vi "Telnet_Init_Challenge_v2.vi"(2 "Max_trials":i32=10, 3 "Address":string="192.168.10.152") -> (0 "connection ID out":refnum<k5>, 1 "telnet_status":bool)   [LabVIEW 2018]
panel:
  out "conn_status":bool
  out "string out":string
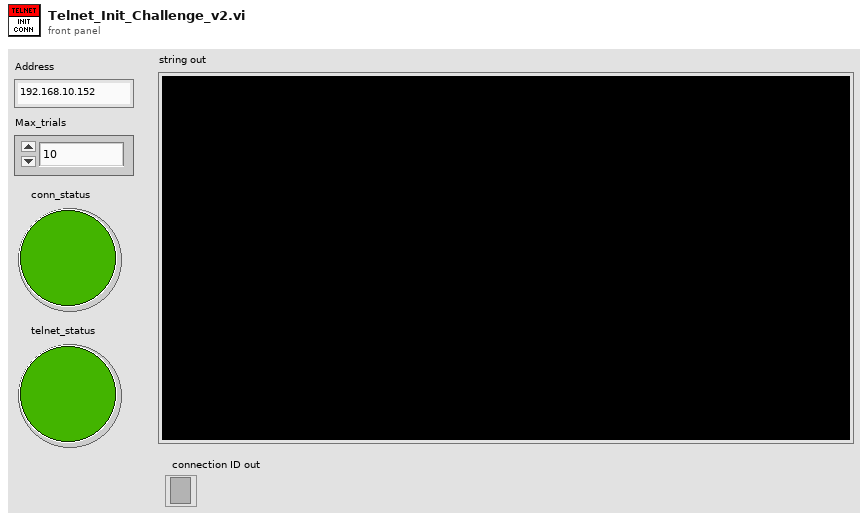
[diagram p1: front panel]
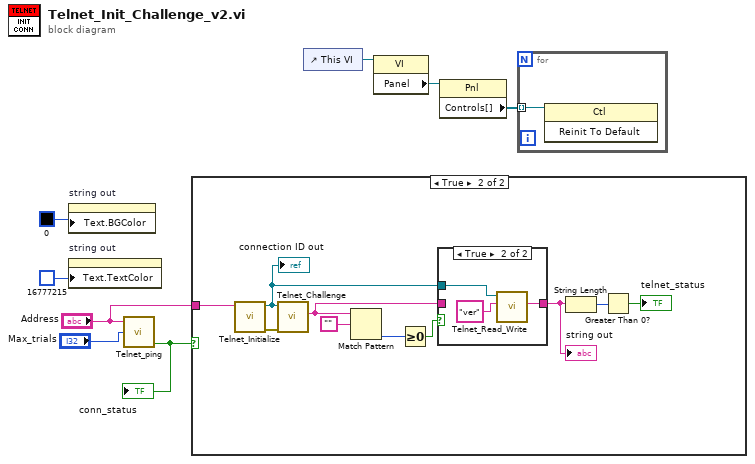
[diagram p0: block diagram]
diagram:
  n1 = property on="string out" class="Str"("Text.BGColor"=u32 0) -> ()  [unwired: 2 in, 2 out]
  n2 = property on="string out" class="Str"("Text.TextColor"=u32 16777215) -> ()  [unwired: 2 in, 2 out]
  n3 = call "Telnet_ping.vi"("Max_trials"="Max_trials", "Address"="Address") -> ("conn_status"=w7:bool)  [unwired: 3 in]
  "conn_status" <- w7
  n4 = case shown="True" w7 {
    tunnel: "Address" -> [_ w17]
    frame False {
    }
    frame True {
      n5 = call "Telnet_Initialize.vi"("Address"=w17) -> ("error out"=w18:errorcluster, "connection ID out"=w9:refnum<k5>)  [unwired: 9 in]
      "connection ID out" <- w9
      n6 = call "Telnet_Challenge.vi"("error in (no error)"=w18, "connection ID in"=w9) -> ("Challenge status"=w12:string)  [unwired: 7 in, 2 out]
      n7 = Match Pattern(string=w12, regular expression="") -> (offset past match=w15:i32)  [unwired: 1 in, 3 out]
      n8 = Greater Or Equal To 0?(x=w15) -> (x >= 0?=w14:bool)
      n9 = case shown="True" w14 {
        tunnel: [w19 w21] -> w11
        tunnel: w9 -> [_ w20]
        tunnel: w12 -> [w19 _]
        frame False {
        }
        frame True {
          n10 = call "Telnet_Read_Write.vi"("Write Telnet Command"="ver", "connection ID"=w20) -> ("string out"=w21:string)  [unwired: 8 in, 1 out]
        }
      }
      "string out" <- w11
      n11 = String Length(string=w11) -> (length=w13:i32)
      n12 = Greater Than 0?(x=w13) -> (x > 0?=→"telnet_status":bool)
    }
  }
  n13 = control-ref of="This VI"() -> (w4:refnum<vi>)
  n14 = property class="VI"(reference=w4) -> ("Panel"=w3:refnum<vi>)  [unwired: 1 in, 2 out]
  n15 = property class="Pnl"(reference=w3) -> ("Controls[]"=w2:refnum<vi>[])  [unwired: 1 in, 2 out]
  n16 = for {
    tunnel: w2 -> [w23] mode=indexing
    n17 = invoke class="Ctl" method="Reinit To Default"(reference=w23) -> ()  [unwired: 2 in, 3 out]
  }
